vi "Available DMA FG.vi"(8 "error in (no error)":errorcluster, 11 "Item Ref":T4 format="%.0x") -> (0 "error out":errorcluster, 2 "Available DMA":T1[](array[typedef]), 3 "Item Ref out":T4=18446744073709551615 format="%.0x")   [LabVIEW 2016, in "FPGA Addon Shared.lvlib"]
uses:
  FPGA Addon Shared.lvlib
  <vilib>/NI Veristand/Custom Device API/Custom Device Item Ref.ctl
  <vilib>/rvi/FIFO/Fifo_Types/Fifo_DMA_Config.ctl
  <vilib>/rvi/DataTransferAndStorage/Container/Common/niFpgaDataTypeControl.ctl
  <vilib>/rvi/ClientSDK/Core/ModuleGeneration/CommunicationInterfaceUtility/niFpgaDmaChannelImplementation.ctl
  <vilib>/NI VeriStand/Custom Device API/Custom Device API.lvlib
  VeriStand-FPGA-Resource-Manager/Source/FPGA Resource Manager System Definition.lvlib
  System Explorer/FPGA Addon System Explorer.lvlib
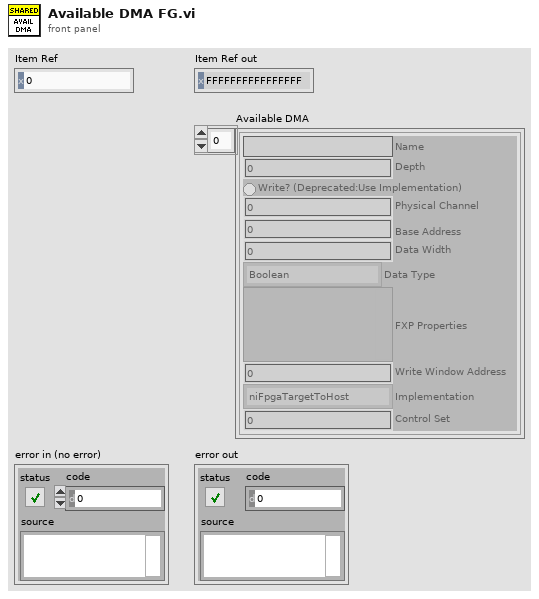
[diagram p1: front panel]
types:
  T1 = typedef "Fifo_DMA_Config.ctl" = cluster{"Name":string, "Depth":u32, "Write? (Deprecated:Use Implementation)":bool, "Physical Channel":u32, "Base Address":u32, "Data Width":u32, "Data Type":T2, "FXP Properties":variant, "Write Window Address":u32, "Implementation":T3, "Control Set":u32}
  T2 = typedef "niFpgaDataTypeControl.ctl" = enum32{"Boolean", "I8", "I16", "I32", "I64", "U8", "U16", "U32", "U64", "FXP", "CustomControl", "SGL"}
  T3 = typedef "niFpgaDmaChannelImplementation.ctl" = enum16{"niFpgaTargetToHost", "niFpgaHostToTarget", "niFpgaPeerToPeerWriter", "niFpgaPeerToPeerReader", "niCoreTargetToHost", "niCoreHostToTarget"}
  T4 = typedef "Custom Device API.lvlib/Custom Device Item Ref.ctl" = u64
  T5 = typedef "Custom Device API.lvlib/Custom Device Item Info.ctl" = cluster{"Name":string, "Is Channel":bool, "GUID":string, "Is Waveform":bool}
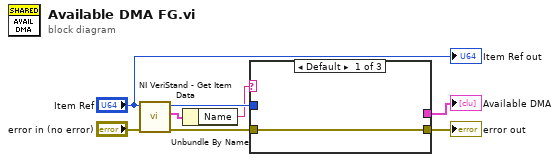
[diagram p0: block diagram]
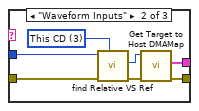
[diagram p2: hidden frame]
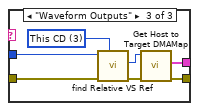
[diagram p3: hidden frame]
diagram:
  n1 = call <vilib>:"NI VeriStand - Get Item Data.vi"("error in (no error)"="error in (no error)", "Item Ref in"="Item Ref") -> ("error out"=w6:errorcluster, "Item Info"=w8:T5, "Item Ref out"=w7:T4)  [unwired: 6 in, 1 out]
  n2 = Unbundle By Name(w8) -> ("Name"=w2:string)
  n3 = case shown="Default" w2 {
    tunnel: w7 -> [_ w16 w23]
    tunnel: w6 -> [w9 w12 w19]
    tunnel: [_ w11 w17] -> w5
    tunnel: [w9 w10 w18] -> w1
    frame Default {
    }
    frame "Waveform Inputs" {
      w15 = u16 3 items=["Targets", "Controller", "Custom Devices", "This CD", "This CD/Group", "This CD/Group/SubGroup"] ("Relative Type")
      n4 = call "find Relative VS Ref.vi"("Relative Type"=w15, "error in (no error)"=w12, "Item Ref in"=w16) -> ("error out"=w13:errorcluster, "Relative Item Ref Out"=w14:T4)  [unwired: 4 in, 3 out]
      n5 = call "Get Target to Host DMAMap.vi"("error in (no error)"=w13, "Item Ref in"=w14) -> ("error out"=w10:errorcluster, "DMA configuration array"=w11:T1[])  [unwired: 7 in, 1 out]
    }
    frame "Waveform Outputs" {
      w22 = u16 3 items=["Targets", "Controller", "Custom Devices", "This CD", "This CD/Group", "This CD/Group/SubGroup"] ("Relative Type")
      n6 = call "find Relative VS Ref.vi"("Relative Type"=w22, "error in (no error)"=w19, "Item Ref in"=w23) -> ("error out"=w20:errorcluster, "Relative Item Ref Out"=w21:T4)  [unwired: 4 in, 3 out]
      n7 = call "Get Host to Target DMAMap.vi"("error in (no error)"=w20, "Item Ref in"=w21) -> ("error out"=w18:errorcluster, "DMA configuration array"=w17:T1[])  [unwired: 7 in, 1 out]
    }
  }
  "error out" <- w1
  "Available DMA" <- w5
  "Item Ref out" <- "Item Ref"
